vi "AlternativeLauncher.vi"() -> ()   [LabVIEW 2013]
panel:
  out "2nd letter":string
  out "1st letter":string
  out "PASSWORD":string
  out "2nd":bool
  out "1st":bool
  out "Input Signal Energy":dbl
  out "Utterance":dbl[](graph)
  out "Slide":i32(slide) scale=0.0..3000.0
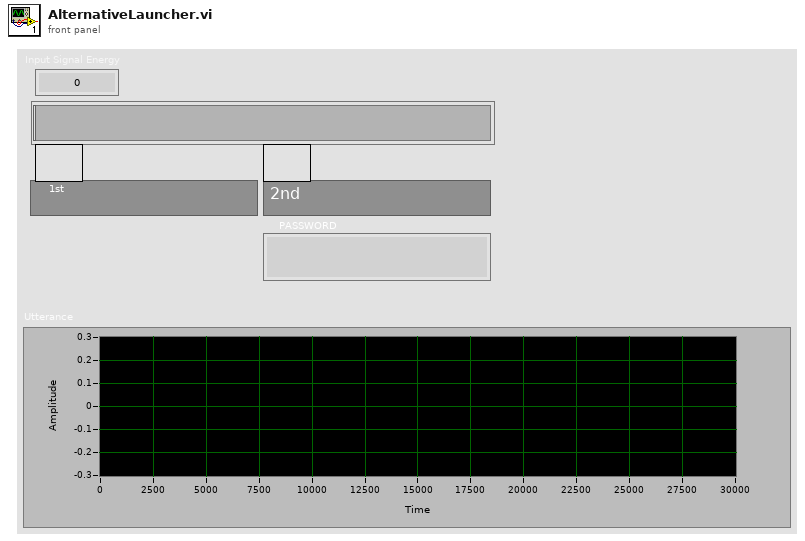
[diagram p1: front panel]
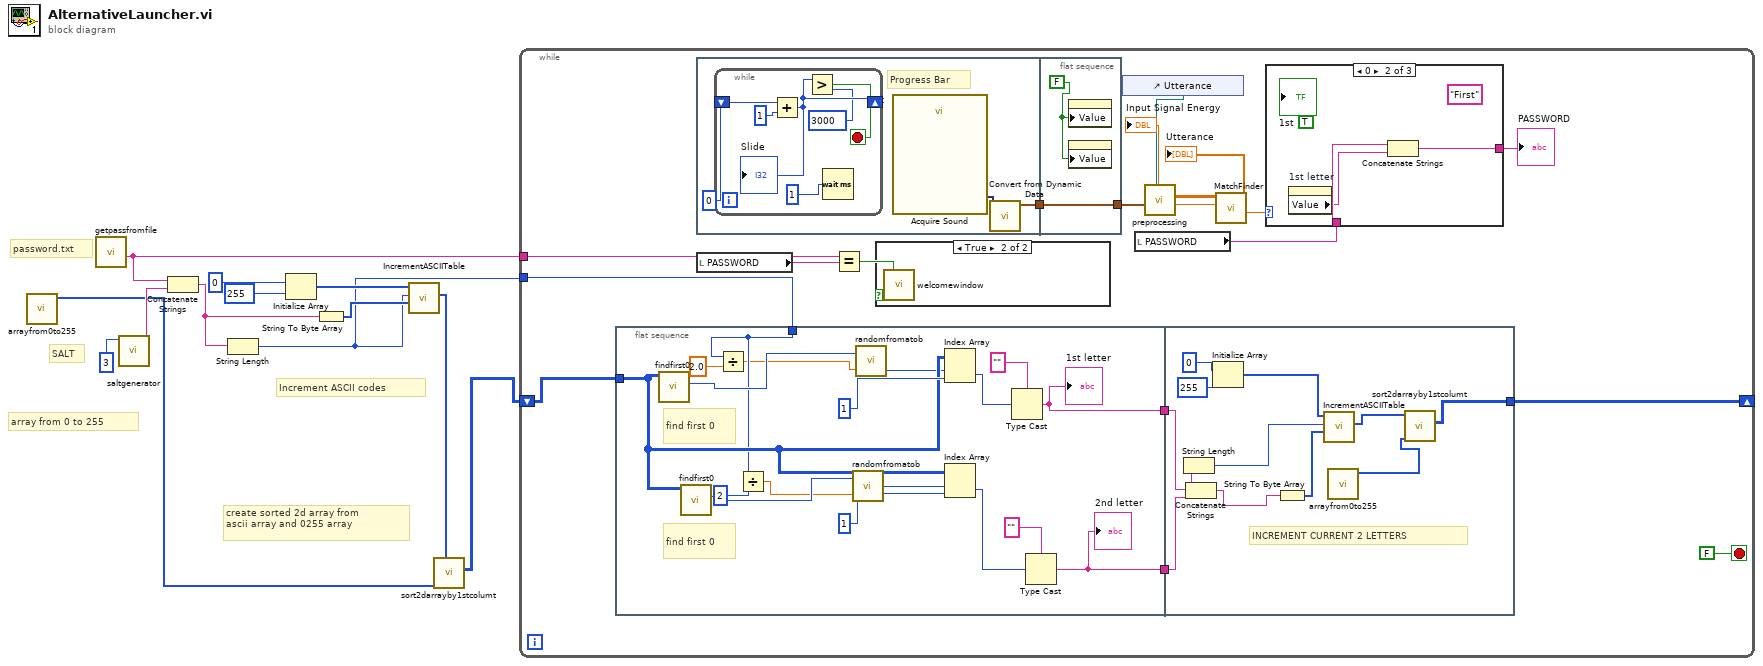
[diagram p0: block diagram]
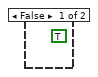
[diagram p2: hidden frame]
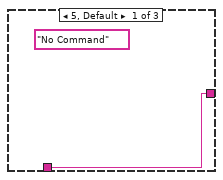
[diagram p3: hidden frame]
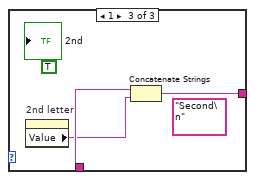
[diagram p4: hidden frame]
diagram:
  # "array from 0 to 255"
  # "create sorted 2d array from \nascii array and 0255 array"
  # "Increment ASCII codes"
  # "SALT"
  # "password.txt"
  n1 = call "arrayfrom0to255.vi"() -> ("Array 2"=w3:i32[])  [unwired: 11 in]
  n2 = call "getpassfromfile.vi"() -> ("line string"=w11:string)  [unwired: 11 in]
  n3 = call "saltgenerator.vi"("Numeric"=3) -> ("string"=w10:string)  [unwired: 10 in]
  n4 = Concatenate Strings(w11, w10) -> (w6:string)
  n5 = String Length(string=w6) -> (length=w1:i32)
  n6 = Initialize Array(0 ("dimension size"), 255 ("dimension size")) -> (w4:i32[])
  n7 = String To Byte Array(string=w6) -> (unsigned byte array=w5:u8[])
  n8 = call "IncrementASCIITable.vi"("0255array"=w5, "Numeric"=w1, "Array in"=w4) -> ("we array"=w9:i32[])  [unwired: 7 in, 1 out]
  n9 = call "sort2darrayby1stcolumt.vi"("array"=w3, "we array"=w9) -> ("Array"=w2:i32[][])  [unwired: 9 in]
  n10 = while {
    tunnel: w11 -> [w20]
    shift-right: [w14] -> _
    shift-left: w2 -> [w15]
    tunnel: w1 -> [w13]
    stop <- FALSE stop-if-true
    n11 = flat-sequence {
      tunnel: w15 -> [w47]
      tunnel: [w42] -> w17
      tunnel: [w41] -> w16
      tunnel: w13 -> [w37]
      tunnel: w17 -> [w55]
      tunnel: w16 -> [w54]
      tunnel: [w50] -> w14
      frame #0 {
        # "find first 0"
        # "find first 0"
        n12 = call "findfirst0.vi"("Array"=w47) -> ("index of element"=w39:i32)  [unwired: 10 in]
        n13 = call "findfirst0.vi"("Array"=w47) -> ("index of element"=w34:i32)  [unwired: 10 in]
        n14 = Divide(x=w37, y=2.0) -> (x/y=w32:dbl)
        n15 = Divide(x=w37, y=2) -> (x/y=w33:dbl)
        n16 = call "randomfromatob.vi"("High (1)"=w34, "Low (0)"=w33) -> ("Random #"=w35:i32)  [unwired: 3 in]
        n17 = call "randomfromatob.vi"("High (1)"=w39, "Low (0)"=w32) -> ("Random #"=w40:i32)  [unwired: 3 in]
        n18 = Index Array(array=w47, index (row)=w40, index (col)=1 ("index (row)")) -> (element=w43:i32)
        n19 = Index Array(array=w47, index (row)=w35, index (col)=1 ("index (row)")) -> (element=w45:i32)
        n20 = Type Cast(type="", x=w43) -> (*(type *) &x=w42:string)
        "1st letter" <- w42
        n21 = Type Cast(type="", x=w45) -> (*(type *) &x=w41:string)
        "2nd letter" <- w41
      }
      frame #1 {
        # "INCREMENT CURRENT 2 LETTERS"
        n22 = Concatenate Strings(w55, w54) -> (w53:string)
        n23 = String Length(string=w53) -> (length=w57:i32)
        n24 = Initialize Array(0 ("dimension size"), 255 ("dimension size")) -> (w58:i32[])
        n25 = String To Byte Array(string=w53) -> (unsigned byte array=w56:u8[])
        n26 = call "IncrementASCIITable.vi"("0255array"=w56, "Numeric"=w57, "Array in"=w58) -> ("we array"=w52:i32[])  [unwired: 7 in, 1 out]
        n27 = call "arrayfrom0to255.vi"() -> ("Array 2"=w51:i32[])  [unwired: 11 in]
        n28 = call "sort2darrayby1stcolumt.vi"("array"=w51, "we array"=w52) -> ("Array"=w50:i32[][])  [unwired: 9 in]
      }
    }
    n29 = flat-sequence {
      tunnel: [w70] -> w25
      tunnel: [w80] -> w26
      tunnel: w25 -> [w80]
      frame #0 {
        # "Progress Bar"
        n30 = while {
          shift-right: [w75] -> _
          shift-left: 0 -> [w78]
          stop <- w73 stop-if-true
          n31 = Add(x=w78, y=1) -> (x+y=w75:i32)
          "Slide" <- w75
          n32 = Greater?(x=w75, y=u32 3000) -> (0:w73:bool)
          n33 = Wait (ms)(milliseconds to wait=u32 1) -> ()  [unwired: 1 out]
        }
        n34 = call "Acquire Sound"() -> ("Data"=w71:dynamicdata)  [unwired: 18 in, 1 out]
        n35 = call "Convert from Dynamic Data"("Dynamic Data Type"=w71) -> ("Array of Waveform"=w70:waveform(dbl)[])  [unwired: 3 in]
      }
      frame #1 {
        w79 = FALSE ("1st")
        n36 = property class="Bool (strict)"("Value"=w79) -> ()  [unwired: 2 in, 2 out]
        n37 = property class="Bool (strict)"("Value"=w79) -> ()  [unwired: 2 in, 2 out]
      }
    }
    n38 = local read "PASSWORD"() -> (w21:string)
    n39 = Equal?(x=w20, y=w21) -> (x = y?=w19:bool)
    n40 = case shown="True" w19 {
      frame False {
        (unwired) TRUE ("Boolean 2")
      }
      frame True {
        n41 = call "welcomewindow.vi"() -> ()  [unwired: 12 in]
      }
    }
    n42 = control-ref of="Utterance"() -> (w28:refnum<vi>)
    n43 = local read "PASSWORD"() -> (w22:string)
    n44 = call "preprocessing.vi"("WaveformGraph in"=w28, "Input Speech"=w26) -> ("Start index"=w31:dbl, "Frames"=w30:dbl[][], "Signal energy"=→"Input Signal Energy":dbl)  [unwired: 6 in, 1 out]
    n45 = call "MatchFinder.vi"("Start index"=w31, "Frames"=w30) -> ("Best Match"=w24:dbl, "Utterance"=→"Utterance":dbl[])  [unwired: 8 in]
    n46 = case shown="0" w24 {
      tunnel: [w61 w64 w68] -> w23
      tunnel: w22 -> [w61 w63 w67]
      frame 5, Default {
        (unwired) "No Command" ("Command")
      }
      frame 0 {
        (unwired) "First" ("Command")
        n47 = property on="1st letter" class="Str"() -> ("Value"=w62:string)  [unwired: 2 in, 2 out]
        n48 = Concatenate Strings(w63, w62) -> (w64:string)
        "1st" <- TRUE ("RIGHT")
      }
      frame 1 {
        (unwired) "Second\n" ("Command")
        n49 = property on="2nd letter" class="Str"() -> ("Value"=w66:string)  [unwired: 2 in, 2 out]
        n50 = Concatenate Strings(w67, w66) -> (w68:string)
        "2nd" <- TRUE ("RIGHT")
      }
    }
    "PASSWORD" <- w23
  }
